vi "Update AO Parameter.vi"(6 "Parameter":T1(ring), 8 "error in":errorcluster, 9 "Value":variant, 10 "Channel":i32, 11 "Instrument.Lockin":refnum<class "Instrument.Lockin.lvclass">) -> (0 "error out":errorcluster, 3 "Instrument.Lockin out":refnum<class "Instrument.Lockin.lvclass">)   [LabVIEW 2019, in "Instrument.Lockin.lvclass"]
uses:
  Instrument.Lockin.lvclass
  Instrument.Lockin.lvclass/Instrument.Lockin.ctl
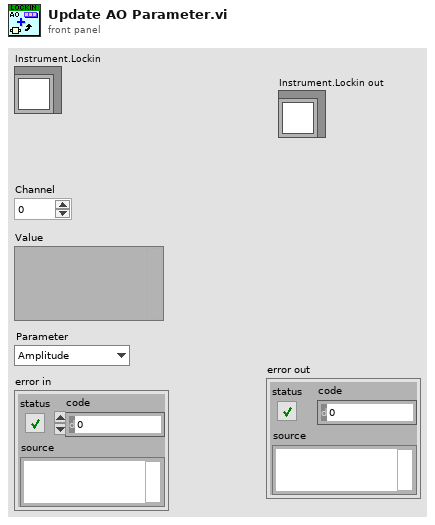
[diagram p1: front panel]
types:
  T1 = enum16{"Amplitude", "DC", "Frequency", "Phase", "Function"}
  T2 = typedef "Instrument.DAQ.lvclass/AO.Channel--Cluster--Array.ctl" = T3[]
  T3 = typedef "Instrument.DAQ.lvclass/AO.Channel--Cluster.ctl" = cluster{"Enable?":bool, "Channel":i32, "Amplitude":dbl, "Offset":dbl, "Frequency":dbl, "Phase":dbl, "Function":T4, "Sweeping?":bool}
  T4 = typedef "Instrument.DAQ.lvclass/AO.Channel.Function--Enum.ctl" = enum16{"Sine", "Triangle", "Square"}
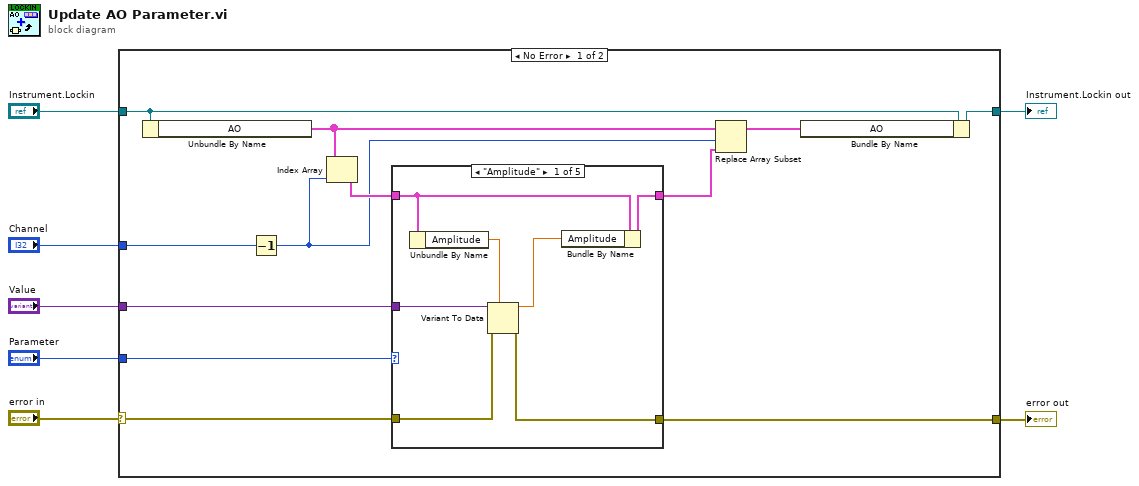
[diagram p0: block diagram]
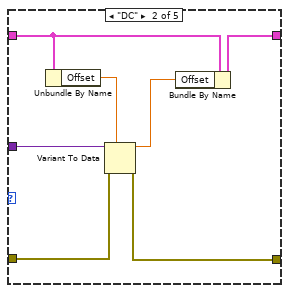
[diagram p2: hidden frame]
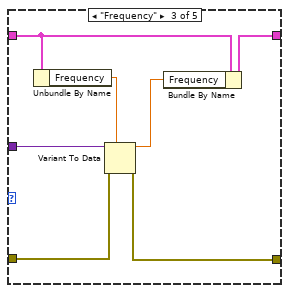
[diagram p3: hidden frame]
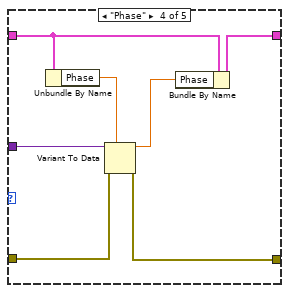
[diagram p4: hidden frame]
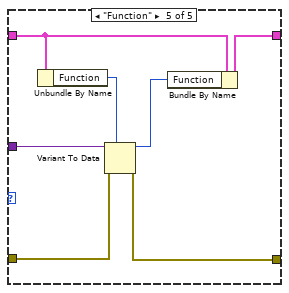
[diagram p5: hidden frame]
diagram:
  n1 = case shown="No Error" "error in" {
    selector: "error in" -> [w8 w56]
    tunnel: "Channel" -> [w19 _]
    tunnel: "Value" -> [w18 _]
    tunnel: [w17 w56] -> w5
    tunnel: "Parameter" -> [w15 _]
    tunnel: "Instrument.Lockin" -> [w11 w55]
    tunnel: [w10 w55] -> w2
    frame No Error {
      n2 = Unbundle By Name(w11) -> ("AO"=w12:T2)
      n3 = Decrement(x=w19) -> (x-1=w13:i32)
      n4 = Index Array(array=w12, index=w13) -> (element=w14:T3)
      n5 = case shown="\"Amplitude\"" w15 {
        tunnel: w14 -> [w26 w33 w40 w47 w54]
        tunnel: w8 -> [w21 w28 w35 w42 w49]
        tunnel: w18 -> [w23 w30 w37 w44 w51]
        tunnel: [w20 w27 w34 w41 w48] -> w17
        tunnel: [w22 w29 w36 w43 w50] -> w16
        frame "Amplitude" {
          n6 = Unbundle By Name(w26) -> ("Amplitude"=w25:dbl)
          n7 = Variant To Data(error in=w21, type=w25, Variant=w23) -> (data=w24:dbl, error out=w20:errorcluster)
          n8 = Bundle By Name(cluster=w26, "Amplitude"=w24) -> (w22:T3)
        }
        frame "DC" {
          n9 = Unbundle By Name(w33) -> ("Offset"=w32:dbl)
          n10 = Variant To Data(error in=w28, type=w32, Variant=w30) -> (data=w31:dbl, error out=w27:errorcluster)
          n11 = Bundle By Name(cluster=w33, "Offset"=w31) -> (w29:T3)
        }
        frame "Frequency" {
          n12 = Unbundle By Name(w40) -> ("Frequency"=w39:dbl)
          n13 = Variant To Data(error in=w35, type=w39, Variant=w37) -> (data=w38:dbl, error out=w34:errorcluster)
          n14 = Bundle By Name(cluster=w40, "Frequency"=w38) -> (w36:T3)
        }
        frame "Phase" {
          n15 = Unbundle By Name(w47) -> ("Phase"=w46:dbl)
          n16 = Variant To Data(error in=w42, type=w46, Variant=w44) -> (data=w45:dbl, error out=w41:errorcluster)
          n17 = Bundle By Name(cluster=w47, "Phase"=w45) -> (w43:T3)
        }
        frame "Function" {
          n18 = Unbundle By Name(w54) -> ("Function"=w53:T4)
          n19 = Variant To Data(error in=w49, type=w53, Variant=w51) -> (data=w52:T4, error out=w48:errorcluster)
          n20 = Bundle By Name(cluster=w54, "Function"=w52) -> (w50:T3)
        }
      }
      n21 = Replace Array Subset(array=w12, new element=w16, index=w13) -> (w9:T2)
      n22 = Bundle By Name(cluster=w11, "AO"=w9) -> (w10:refnum<class "Instrument.Lockin.lvclass">)
    }
    frame Error {
    }
  }
  "Instrument.Lockin out" <- w2
  "error out" <- w5
